vi "Disconnect.vi"(8 "error in (no error)":errorcluster, 11 "2230G in":refnum<class "2230G.lvclass">) -> (0 "error out":errorcluster, 3 "2230G out":refnum<class "2230G.lvclass">)   [LabVIEW 2018, in "2230G.lvlib" / "2230G.lvclass"]
uses:
  2230G.lvclass
  <instrlib>/Keithley KE22xx Series/Keithley KE22xx Series.lvlib
  PPLs/Power Supply/Parent/Power_Supply.lvlibp/Power Supply.lvclass
  C:/Projects/LabVIEW/PPLs/Power Supply/Parent/Power_Supply.lvlibp/Power Supply.lvclass
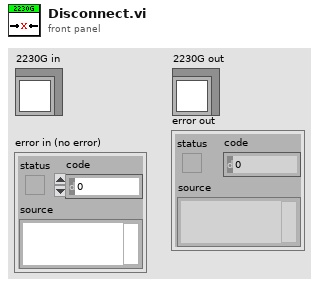
[diagram p1: front panel]
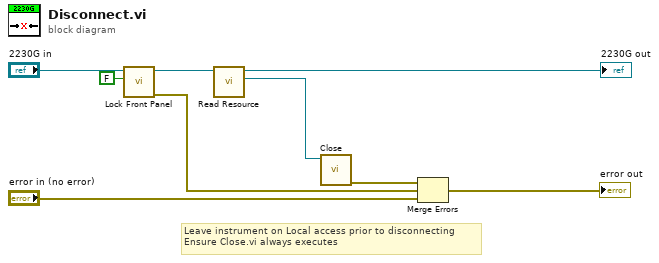
[diagram p0: block diagram]
diagram:
  # "Leave instrument on Local access prior to disconnecting\nEnsure Close.vi always executes"
  n1 = call-dynamic "Lock Front Panel.vi"("Lock?"=FALSE, "2230G in"="2230G in") -> ("error out"=w2:errorcluster, "2230G out"=w3:refnum<class "2230G.lvclass">)  [unwired: 8 in]
  n2 = call "Read Resource.vi"("Power Supply in"=w3) -> ("Resource"=w5:refnum<visa-resource-name>, "Power Supply out"=→"2230G out":refnum<class "2230G.lvclass">)  [unwired: 8 in, 1 out]
  n3 = call <instrlib>:"Close.vi"("VISA resource name"=w5) -> ("error out"=w9:errorcluster)  [unwired: 10 in]
  n4 = Merge Errors(w9, w2, "error in (no error)") -> (→"error out":errorcluster)
